vi "SPL Calculator (2).vi"(8 "Error In":errorcluster, 9 "Gain":dbl(slide) min=0.0 max=50.0 scale=0.0..50.0, 10 "Microphone Sensitvity (dBV/Pa)":dbl format="%#_13g", 11 "Filtered Signal":dynamicdata(waveform)) -> (0 "Error Out":errorcluster, 3 "SPL":dbl)   [LabVIEW 2020, in "CollectionSupport.lvlib"]
uses:
  CollectionSupport.lvlib
  <vilib>/measure/madcrms.llb/Basic Averaged DC-RMS for 1 Chan.vi
  <vilib>/measure/NI_MAPro.lvlib
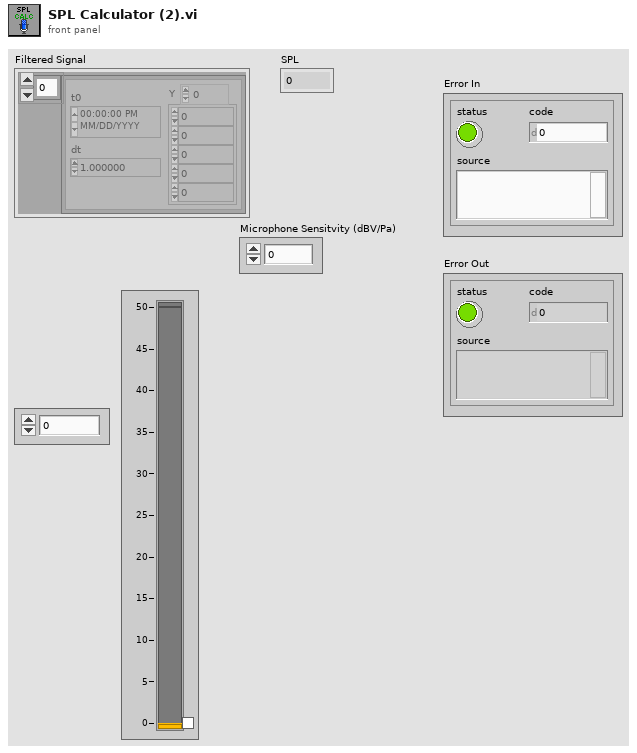
[diagram p1: front panel]
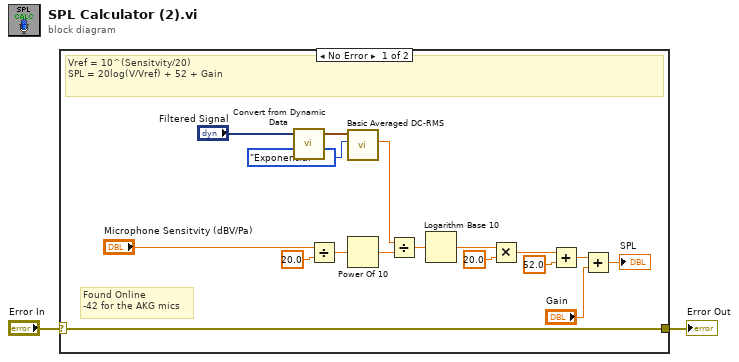
[diagram p0: block diagram]
diagram:
  n1 = case shown="No Error" "Error In" {
    selector: "Error In" -> [w3 w20]
    tunnel: [w3 w20] -> w1
    frame No Error {
      # "Found Online\n-42 for the AKG mics"
      # "Vref = 10^(Sensitvity/20)\nSPL = 20log(V/Vref) + 52 + Gain"
      n2 = call "Convert from Dynamic Data"("Dynamic Data Type"="Filtered Signal") -> ("Waveform"=w16:waveform(dbl))  [unwired: 3 in]
      n3 = Divide(x="Microphone Sensitvity (dBV/Pa)", y=20.0) -> (x/y=w5:dbl)
      n4 = call-poly <vilib>:"Basic Averaged DC-RMS.vi"("averaging type"=enum16{"Linear", "Exponential"}."Exponential", "signal in"=w16) -> ("RMS value"=w15:dbl)  [unwired: 6 in, 3 out]
      n5 = Power Of 10(x=w5) -> (10^x=w4:dbl)
      n6 = Divide(x=w15, y=w4) -> (x/y=w14:dbl)
      n7 = Logarithm Base 10(1:w14) -> (0:w13:dbl)
      n8 = Multiply(x=w13, y=20.0) -> (x*y=w10:dbl)
      n9 = Add(x=w10, y=52.0) -> (x+y=w9:dbl)
      n10 = Add(x=w9, y="Gain") -> (x+y=→"SPL":dbl)
    }
    frame Error {
    }
  }
  "Error Out" <- w1
